vi "Draw Compass Picture.vi"(7 "draw options":T1={"Outer Border Color"=0, "Inner Border Color"=6316128, "Outer Gradient Color"=2565927, "Inner Gradient Color"=16860, "Compass North Pointer Color"=16711680, "Compass Pointer Color 1"=13355429, "Compass Pointer Color 2"=14934973, "Direction Pointer Color"=16765184, "Text Box Outline Color"=13355429, "Text Box Background Color"=14934973, "Scale Color"=16448250, "Text Color"=0, "Draw Gradient"=TRUE, "Draw Rose"=TRUE, "Simple Scale"=TRUE, "Draw Text"=FALSE, "Font Name"="Helvetica", "Angle Units"=enum."Degrees"}, 8 "error in (no error)":errorcluster, 9 "DrawAreaSize":T3={"Width"=100, "Height"=100}, 10 "angle":dbl, 11 "picture in":picture) -> (0 "error out":errorcluster, 3 "picture out":picture)   [LabVIEW 2017, in "NI_Robotics_Compass Picture.lvlib"]
uses:
  <vilib>/robotics/Controls/Compass Indicator/Compass Picture/NI_Robotics_Compass Picture.lvlib
  <vilib>/Utility/miscctls.llb/LVBoundsTypeDef.ctl
  <vilib>/robotics/Controls/Compass Indicator/Compass Picture/Draw Options.ctl
  <vilib>/robotics/Controls/Utilities/Angle Units.ctl
  <vilib>/robotics/Controls/Compass Indicator/Compass Picture/Draw Area State.ctl
  <vilib>/Analysis/coordinate.llb/Wrap Angle.vi
  <vilib>/Analysis/coordinate.llb/Wrap Angle (scalar).vi
  <vilib>/robotics/Controls/Utilities/Fit Font Size to Box.vi
  <vilib>/robotics/Controls/Compass Indicator/Compass Picture/Build Text.vi
  <vilib>/robotics/Controls/Compass Indicator/Compass Picture/Draw Rose Pointer.vi
  <vilib>/robotics/Controls/Compass Indicator/Compass Picture/Draw Scale Line.vi
  <vilib>/picture/picture.llb/Draw Text at Point.vi
  <vilib>/picture/picture.llb/Draw Rect.vi
  <vilib>/picture/picture.llb/Get Text Rect.vi
  <vilib>/Utility/AngleManip/Radians to Degrees.vi
  <vilib>/Utility/AngleManip/Radians to Degrees (Scalar DBL).vi
  <vilib>/picture/picture.llb/Draw Multiple Lines.vi
  <vilib>/Utility/AngleManip/Degrees to Radians.vi
  <vilib>/Utility/AngleManip/Degrees to Radians (Scalar DBL).vi
  <vilib>/picture/pictutil.llb/Draw Circle by Radius.vi
  <vilib>/picture/pictutil.llb/Hilite Color.vi
  <vilib>/Utility/AngleManip/Degrees to Radians (Array DBL).vi
  <vilib>/Utility/colorconv.llb/RGB to Color.vi
  <vilib>/Utility/colorconv.llb/Color to RGB.vi
  <vilib>/robotics/Controls/Utilities/NI_Robotics_Control Utilities.lvlib
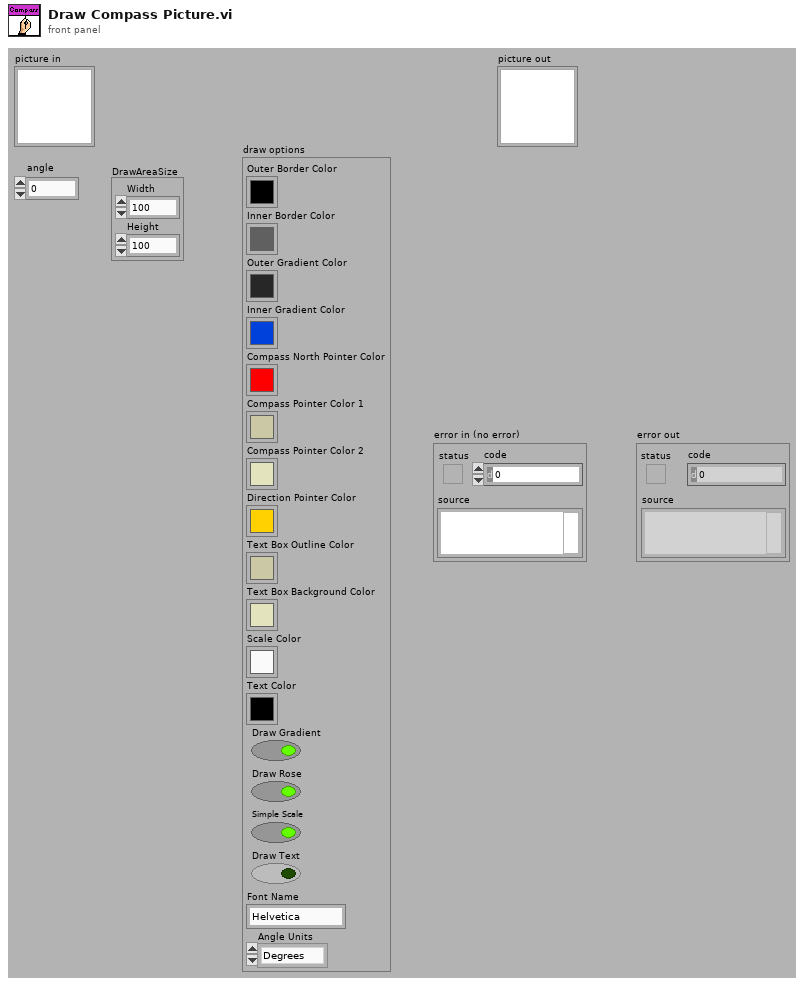
[diagram p1: front panel]
types:
  T1 = typedef "NI_Robotics_Compass Picture.lvlib/Draw Options.ctl" = cluster{"Outer Border Color":u32, "Inner Border Color":u32, "Outer Gradient Color":u32, "Inner Gradient Color":u32, "Compass North Pointer Color":u32, "Compass Pointer Color 1":u32, "Compass Pointer Color 2":u32, "Direction Pointer Color":u32, "Text Box Outline Color":u32, "Text Box Background Color":u32, "Scale Color":u32, "Text Color":u32, "Draw Gradient":bool, "Draw Rose":bool, "Simple Scale":bool, "Draw Text":bool, "Font Name":string, "Angle Units":T2}
  T2 = typedef "NI_Robotics_Control Utilities.lvlib/Angle Units.ctl" = enum16{"Radians", "Degrees"}
  T3 = typedef "LVBoundsTypeDef.ctl" = cluster{"Width":u32, "Height":u32}
  T4 = typedef "NI_Robotics_Compass Picture.lvlib/Draw Area State.ctl" = cluster{"Center":cluster{"horizontal":i16, "vertical":i16}, "Max Radius":dbl, "DrawAreaSize":T3, "Medium Pen":cluster{"Width":u16, "Style":enum32{"Solid", "Dash", "Dot", "DashDot", "DashDotDot"}}, "Thick Pen":cluster{"Width":u16, "Style":enum32{"Solid", "Dash", "Dot", "DashDot", "DashDotDot"}}}
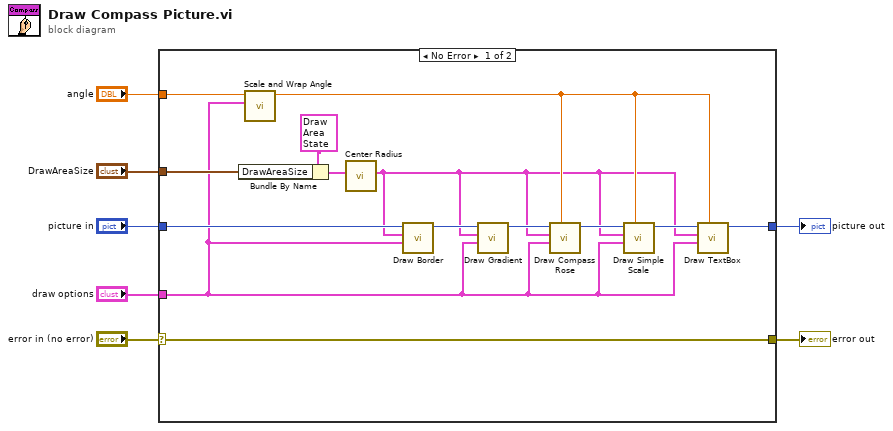
[diagram p0: block diagram]
diagram:
  n1 = case shown="No Error" "error in (no error)" {
    selector: "error in (no error)" -> [w12 w22]
    tunnel: "angle" -> [w11 _]
    tunnel: [w15 w23] -> w6
    tunnel: "DrawAreaSize" -> [w14 _]
    tunnel: "draw options" -> [w8 _]
    tunnel: "picture in" -> [w13 w23]
    tunnel: [w12 w22] -> w1
    frame No Error {
      n2 = Bundle By Name(cluster=T4 {"Center"={"horizontal"=0, "vertical"=0}, "Max Radius"=0.0, "DrawAreaSize"={"Width"=0, "Height"=0}, "Medium Pen"={"Width"=0, "Style"=enum."Solid"}, "Thick Pen"={"Width"=0, "Style"=enum."Solid"}} ("draw area cache in"), "DrawAreaSize"=w14) -> (w20:T4)
      n3 = call <vilib>:"Scale and Wrap Angle.vi"("Draw Options"=w8, "angle"=w11) -> ("angle (rad)"=w10:dbl)  [unwired: 9 in]
      n4 = call <vilib>:"Center Radius.vi"("draw area cache in"=w20) -> ("draw area cache out"=w9:T4)  [unwired: 6 in, 4 out]
      n5 = call <vilib>:"Draw Border.vi"("draw options"=w8, "draw area cache"=w9, "picture in"=w13) -> ("picture out"=w19:picture)  [unwired: 8 in]
      n6 = call <vilib>:"Draw Gradient.vi"("draw options"=w8, "draw area cache in"=w9, "picture in"=w19) -> ("picture out"=w18:picture)  [unwired: 8 in]
      n7 = call <vilib>:"Draw Compass Rose.vi"("heading (rad)"=w10, "draw options"=w8, "draw area cache in"=w9, "picture in"=w18) -> ("picture out"=w17:picture)  [unwired: 7 in]
      n8 = call <vilib>:"Draw Simple Scale.vi"("heading (rad)"=w10, "Draw Options"=w8, "draw area cache"=w9, "picture in"=w17) -> ("picture out"=w16:picture)  [unwired: 7 in]
      n9 = call <vilib>:"Draw TextBox.vi"("heading (rad)"=w10, "draw options"=w8, "draw area cache"=w9, "picture in"=w16) -> ("picture out"=w15:picture)  [unwired: 7 in]
    }
    frame Error {
    }
  }
  "picture out" <- w6
  "error out" <- w1
